vi "OE 4 Butterworth (1).vi"() -> ()   [LabVIEW 2018]
uses:
  <vilib>/Analysis/3filter.llb/Filter Passband Type.ctl
  <vilib>/Analysis/3filter.llb/Butterworth Filter (DBL).vi
  <vilib>/Analysis/NI_AALBase.lvlib
panel:
  in  "enable":bool
  out "Out":dbl[](array[numeric])
  in  "In":dbl[](array[numeric])
  in  "Cutoff Freq.":dbl
  in  "Freq. Bound":dbl
  in  "sampling freq: fs":dbl=1.0 format="%0.2f"
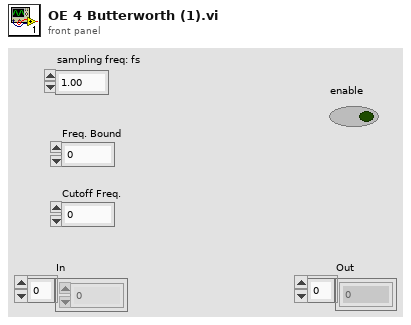
[diagram p1: front panel]
types:
  T1 = typedef "NI_AALBase.lvlib/Filter Passband Type.ctl" = enum32{"Lowpass", "Highpass", "Bandpass", "Bandstop"}
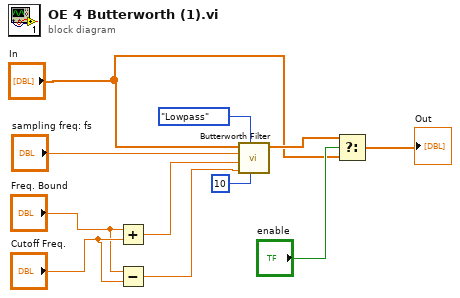
[diagram p0: block diagram]
diagram:
  n1 = Add(x="Freq. Bound", y="Cutoff Freq.") -> (x+y=w8:dbl)
  n2 = Subtract(x="Freq. Bound", y="Cutoff Freq.") -> (x-y=w5:dbl)
  n3 = call-poly <vilib>:"Butterworth Filter.vi"("order"=10, "filter type"=Filter_Passband_Type."Lowpass", "low cutoff freq: fl"=w5, "high cutoff freq: fh"=w8, "sampling freq: fs"="sampling freq: fs", "X"="In") -> ("Filtered X"=w3:dbl[])  [unwired: 2 in, 1 out]
  n4 = Select(t=w3, s="enable", f="In") -> (s? t:f=→"Out":dbl[])
